vi "Read Registry Value String.vi"(8 "error in (no error)":errorcluster, 10 "key":string, 11 "Path":string) -> (0 "error out":errorcluster, 1 "function return":string, 2 "key out":string, 3 "Path out":string)   [LabVIEW 2017, in "LumencorDLLDbg64.lvlib"]
doc: "This function Read the Light Engine Color Map from the Registry.\nOnly use this function if instructed to by Lumencor.\n\n\nextern \"C\" LUMENCORDLL2B_API char * ReadRegistryValueString(char *Path, char *key);"
uses:
  LumencorDLLDbg64.lvlib
  LumencorDLLDbg64.dll
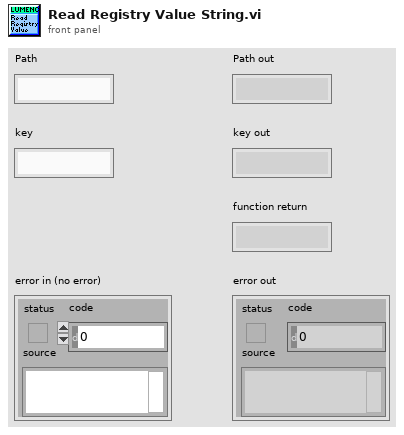
[diagram p1: front panel]
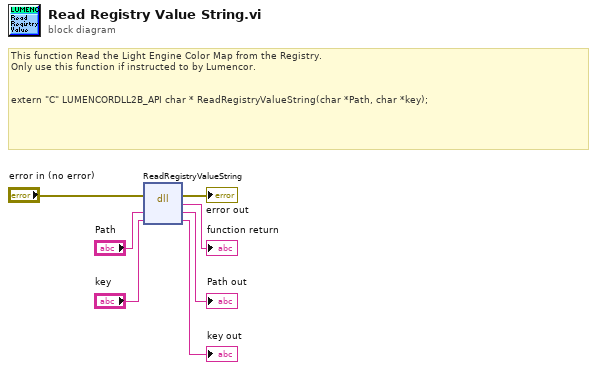
[diagram p0: block diagram]
diagram:
  # "This function Read the Light Engine Color Map from the Registry.\nOnly use this function if instructed to by Lumencor.\n\n\nextern \"C\" LUMENCORDLL2B_API char * ReadRegistryValueString(char *Path, char *key);"
  n1 = dll-call lib="Q:/GIT -- Lumencor DLL4/LabVIEW Library (64bit)/LumencorDLLDbg64.*" fn="ReadRegistryValueString"(error in="error in (no error)", "Path"="Path", "key"="key") -> (error out=→"error out":errorcluster, →"function return":string, "Path"=→"Path out":string, "key"=→"key out":string)  [unwired: 2 in, 1 out]
